vi "Add Turn Stats.vi"(10 "Team Stats":T1, 11 "Team in":refnum<class "Team.lvclass">) -> (3 "Team out":refnum<class "Team.lvclass">)   [LabVIEW 2020, in "SquareBattle.lvlib" / "Team.lvclass"]
uses:
  Team.lvclass
  Team Stats.ctl
  Team.lvclass/Team.ctl
  SquareBattle.lvlib
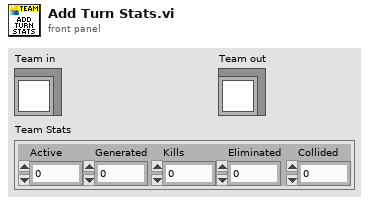
[diagram p1: front panel]
types:
  T1 = typedef "SquareBattle.lvlib/Team Stats.ctl" = cluster{"Active":i32, "Generated":i32, "Kills":i32, "Eliminated":i32, "Collided":i32}
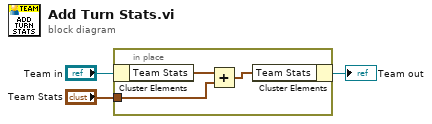
[diagram p0: block diagram]
diagram:
  n1 = in-place {
    in-place-border: "Team Stats" -> [w5]
    n2 = in-place-cluster #1("Team in") -> ("Team Stats"=w6:T1)
    n3 = Add(x=w6, y=w5) -> (x+y=w4:T1)
    n4 = in-place-cluster #1("Team Stats"=w4) -> (→"Team out":refnum<class "Team.lvclass">)
  }
